vi "Perform Action.vi"(8 "error in":errorcluster, 10 "Input":variant, 11 "DAQmx No Op in":refnum<class "DAQmx No Op.lvclass">) -> (0 "error out":errorcluster, 2 "Output":variant, 3 "DAQmx No Op out":refnum<class "DAQmx No Op.lvclass">)   [LabVIEW 2023, in "DAQmx No Op.lvclass"]
uses:
  DAQmx No Op.lvclass
  DAQmx No Op.lvclass/DAQmx No Op.ctl
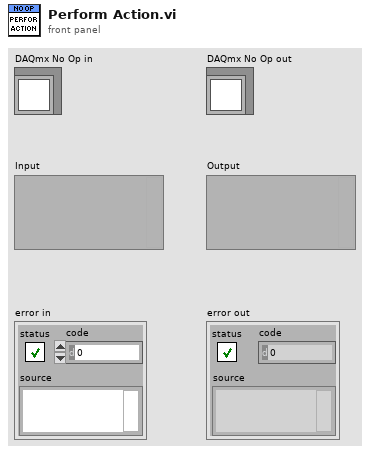
[diagram p1: front panel]
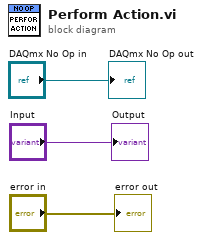
[diagram p0: block diagram]
diagram:
  "error out" <- "error in"
  "DAQmx No Op out" <- "DAQmx No Op in"
  "Output" <- "Input"
